vi "Calc Cmd Numeric.vi"(8 "error in (no error)":errorcluster, 9 "Cmd Value":dbl, 10 "Name":string, 11 "Tare Calc in":refnum<class "Tare Calc.lvclass">) -> (0 "error out":errorcluster, 3 "Tare Calc out":refnum<class "Tare Calc.lvclass">)   [LabVIEW 2020, in "VolatusCalcs.lvlib" / "Tare Calc.lvclass"]
uses:
  Tare Calc.lvclass
  Tare Calc.lvclass/Tare Calc.ctl
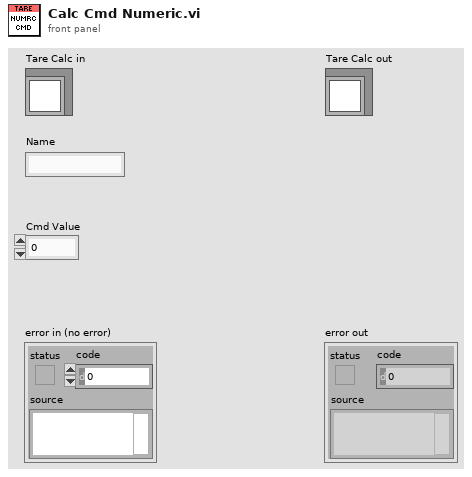
[diagram p1: front panel]
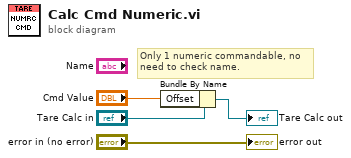
[diagram p0: block diagram]
diagram:
  # "Only 1 numeric commandable, no need to check name."
  n1 = Bundle By Name(cluster="Tare Calc in", "Offset"="Cmd Value") -> (→"Tare Calc out":refnum<class "Tare Calc.lvclass">)
  "error out" <- "error in (no error)"
